vi "BuildSpecExists.vi"(8 "error in":errorcluster, 10 "BuildSpec in":string, 11 "ProjectPath":path) -> (0 "error out":errorcluster, 1 "Build Type":string, 2 "BuildSpec out":string, 3 "ProjectPath dup":path)   [LabVIEW 2020, in "CICD.lvlib"]
doc: "Checks if build spec exists and throws an error if not."
uses:
  CICD.lvlib
  <vilib>/Utility/error.llb/Error Cluster From Error Code.vi
  <vilib>/ErrorRing/Error Ring.xnode
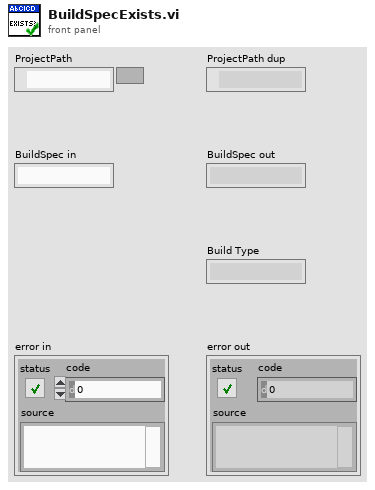
[diagram p1: front panel]
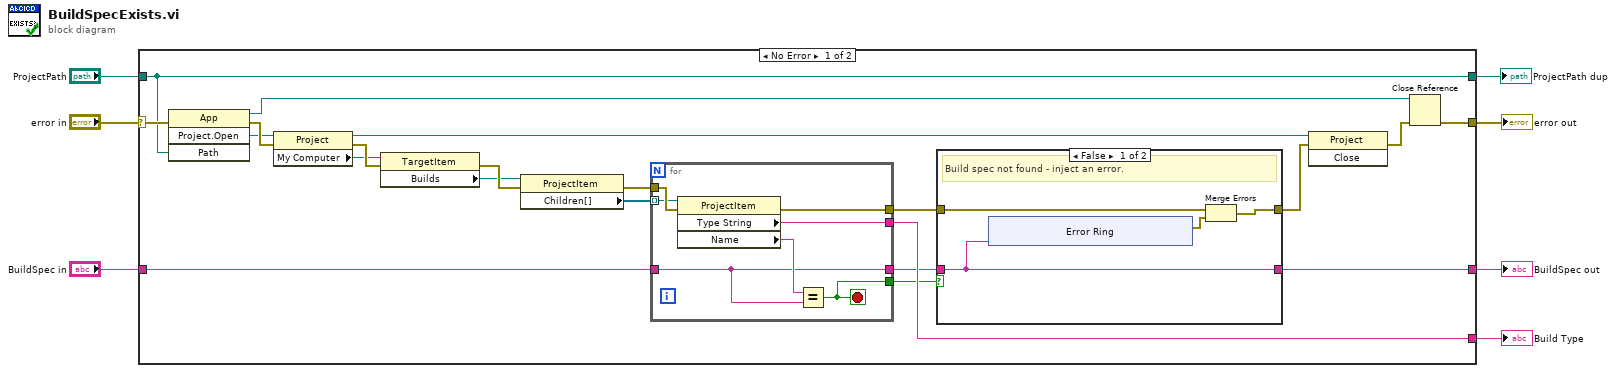
[diagram p0: block diagram]
diagram:
  n1 = case shown="No Error" "error in" {
    selector: "error in" -> [w21 w51]
    tunnel: [w19 _] -> w5
    tunnel: "BuildSpec in" -> [w18 w50]
    tunnel: "ProjectPath" -> [w10 w49]
    tunnel: [w11 w50] -> w2
    tunnel: [w22 w51] -> w7
    tunnel: [w10 w49] -> w1
    frame No Error {
      n2 = invoke class="App" method="Project.Open"(error in=w21, "Path"=w10) -> (reference out=w14:refnum<vi>, error out=w24:errorcluster, "Project:Open"=w15:refnum<vi>)  [unwired: 2 in, 1 out]
      n3 = property class="Project"(reference=w15, error in=w24) -> (reference out=w8:refnum<vi>, error out=w25:errorcluster, "My Computer"=w16:refnum<vi>)
      n4 = property class="TargetItem"(reference=w16, error in=w25) -> (error out=w26:errorcluster, "Builds"=w20:refnum<vi>)  [unwired: 1 out]
      n5 = property class="ProjectItem"(reference=w20, error in=w26) -> (error out=w27:errorcluster, "Children[]"=w17:refnum<vi>[])  [unwired: 1 out]
      n6 = for {
        tunnel: w27 -> [w47]
        tunnel: w17 -> [w46] mode=indexing
        tunnel: [w48] -> w28
        tunnel: w18 -> [w42]
        tunnel: [w45] -> w19
        tunnel: [w44] -> w13
        tunnel: [w42] -> w12
        stop <- w44 stop-if-true
        n7 = property class="ProjectItem"(reference=w46, error in=w47) -> (error out=w48:errorcluster, "Type String"=w45:string, "Name"=w43:string)  [unwired: 1 out]
        n8 = Equal?(x=w43, y=w42) -> (x = y?=w44:bool)
      }
      n9 = case shown="False" w13 {
        tunnel: w28 -> [w32 w41]
        tunnel: [w31 w41] -> w23
        tunnel: w12 -> [w29 w40]
        tunnel: [w29 w40] -> w11
        frame False {
          # "Build spec not found - inject an error."
          n10 = xnode "Error Ring"("parameter 0"=w29) -> ("error out"=w30:errorcluster)
          n11 = Merge Errors(w32, w30) -> (w31:errorcluster)
        }
        frame True {
        }
      }
      n12 = invoke class="Project" method="Close"(reference=w8, error in=w23) -> (error out=w9:errorcluster)  [unwired: 1 in, 2 out]
      n13 = Close Reference(reference=w14, error in (no error)=w9) -> (error out=w22:errorcluster)
    }
    frame Error {
    }
  }
  "BuildSpec out" <- w2
  "Build Type" <- w5
  "error out" <- w7
  "ProjectPath dup" <- w1
